vi "FlatToRichcif_manager_QueryConfigResponse.vi"(5 "OutputClusterType":T1, 11 "InputCluster":T3) -> (3 "OutputCluster":T1)   [LabVIEW 2021, in "CIF_Manager_client.lvlib"]
uses:
  CIF_Manager_client.lvlib
  cif_manager_QueryConfigResponse_Flat.ctl
  cif_manager_FileData_Flat.ctl
  cif_manager_QueryConfigResponse.ctl
  cif_manager_FileData.ctl
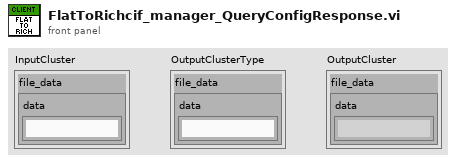
[diagram p1: front panel]
types:
  T1 = typedef "CIF_Manager_client.lvlib/cif_manager_QueryConfigResponse.ctl" = cluster{"file_data":T2}
  T2 = typedef "CIF_Manager_client.lvlib/cif_manager_FileData.ctl" = cluster{"data":string}
  T3 = typedef "CIF_Manager_client.lvlib/cif_manager_QueryConfigResponse_Flat.ctl" = cluster{"file_data":T4}
  T4 = typedef "CIF_Manager_client.lvlib/cif_manager_FileData_Flat.ctl" = cluster{"data":string}
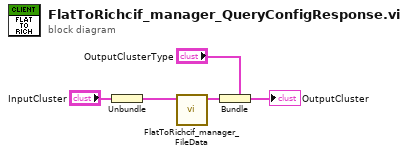
[diagram p0: block diagram]
diagram:
  n1 = Unbundle "Unbundle"("InputCluster") -> ("file_data"=w2:T4)
  n2 = call "FlatToRichcif_manager_FileData.vi"("InputCluster"=w2) -> ("OutputCluster"=w1:T2)  [unwired: 10 in]
  n3 = Bundle "Bundle"(cluster="OutputClusterType", "file_data"=w1) -> (→"OutputCluster":T1)
